vi "CH_LM Calibration Gain-Offset Dialog.vi"(0 "Meter Index":i32, 1 "Probe Type":T1, 5 "error in (no error)":errorcluster, 7 "Timeout / ms (3000)":i32=1000) -> (11 "Lock timed out":bool, 14 "Meter Index":i32, 15 "OK":bool, 16 "Thermopile Calibration":T5, 17 "Pyroelectric Calibration":T2, 18 "Optical Calibration":T4, 19 "error out":errorcluster)   [LabVIEW 2012, in "CH_LM.lvlib"]
doc: "This command stores gain and ADC offset correction data to the meter non-volatile memory. Different correction values are used for each input circuit and gain setting. See the Greenbuster TOP Theory of Operation for more information.\n\n<B>Note:</B> Error 100 will be raised if a valid password has not set since the last power off/on cycle."
uses:
  CH_LM.lvlib
  CH_LM Calibration Data Pyroelectric.ctl
  CH_LM Calibration Data Thermopile.ctl
  CH_LM Calibration Data Optical.ctl
  CH_LM ProbeType.ctl
  CH_LM Calibration Data.ctl
panel:
  in  "Cancel Button":bool
  out "Probe Type":T1
  in  "OK Button":bool
  in  "Optical Calibration":T4
  in  "Thermopile Calibration":T5
  in  "Pyroelectric Calibration":T2
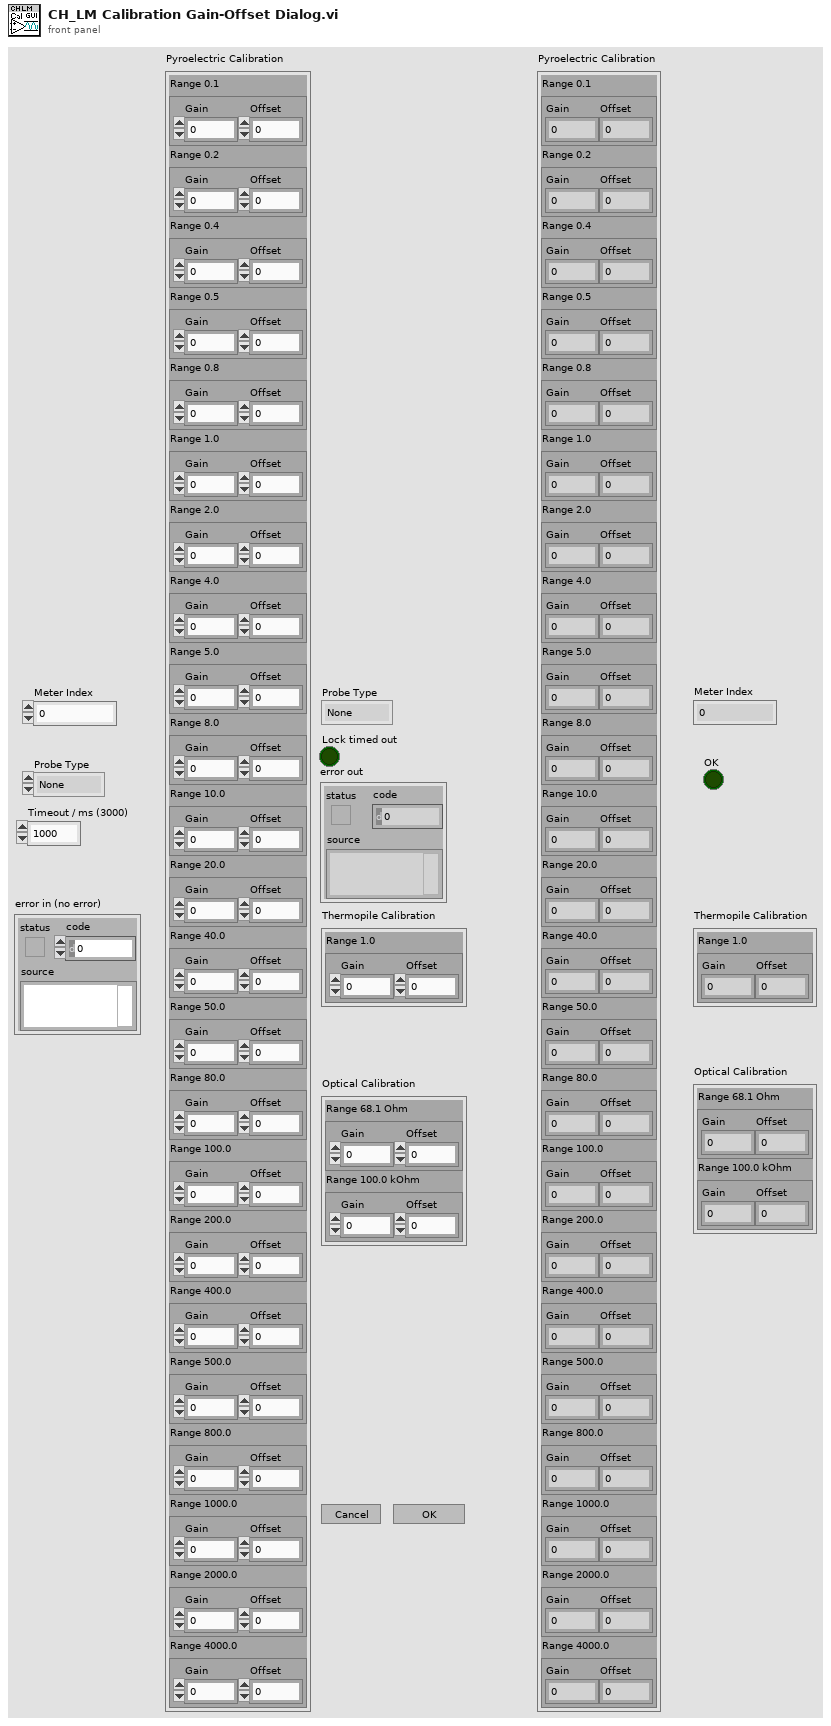
[diagram p1: front panel]
types:
  T1 = typedef "CH_LM.lvlib/CH_LM ProbeType.ctl" = enum16{"None", "Thermopile", "Pyroelectric", "Optical"}
  T2 = typedef "CH_LM.lvlib/CH_LM Calibration Data Pyroelectric.ctl" = cluster{"Range 0.1":T3, "Range 0.2":T3, "Range 0.4":T3, "Range 0.5":T3, "Range 0.8":T3, "Range 1.0":T3, "Range 2.0":T3, "Range 4.0":T3, "Range 5.0":T3, "Range 8.0":T3, "Range 10.0":T3, "Range 20.0":T3, "Range 40.0":T3, "Range 50.0":T3, "Range 80.0":T3, "Range 100.0":T3, "Range 200.0":T3, "Range 400.0":T3, "Range 500.0":T3, "Range 800.0":T3, "Range 1000.0":T3, "Range 2000.0":T3, "Range 4000.0":T3}
  T3 = typedef "CH_LM.lvlib/CH_LM Calibration Data.ctl" = cluster{"Gain":dbl, "Offset":dbl}
  T4 = typedef "CH_LM.lvlib/CH_LM Calibration Data Optical.ctl" = cluster{"Range 68.1 Ohm":T3, "Range 100.0 kOhm":T3}
  T5 = typedef "CH_LM.lvlib/CH_LM Calibration Data Thermopile.ctl" = cluster{"Range 1.0":T3}
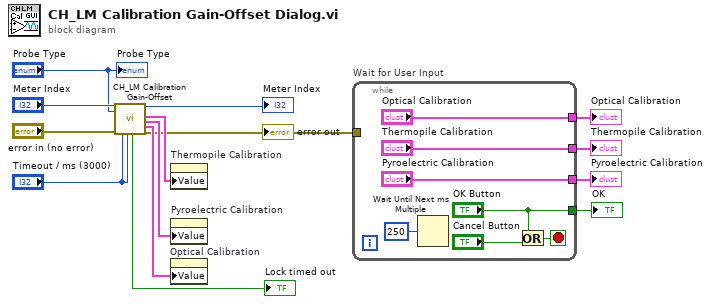
[diagram p0: block diagram]
diagram:
  n1 = call "CH_LM Calibration Gain-Offset.vi"("Meter Index"="Meter Index", "Probe Type"="Probe Type", "error in (no error)"="error in (no error)", "Timeout / ms (3000)"="Timeout / ms (3000)", "Lock Timeout / ms (1000)"="Timeout / ms (3000)") -> ("Lock timed out"=→"Lock timed out":bool, "Meter Index"=→"Meter Index":i32, "Thermopile Calibration"=w8:T5, "Pyroelectric Calibration"=w7:T2, "Optical Calibration"=w6:T4, "error out"=w2:errorcluster)  [unwired: 4 in, 5 out]
  "error out" <- w2
  n2 = property on="Thermopile Calibration" class="Clust (strict)"("Value"=w8) -> ()  [unwired: 2 in, 2 out]
  n3 = property on="Pyroelectric Calibration" class="Clust (strict)"("Value"=w7) -> ()  [unwired: 2 in, 2 out]
  n4 = property on="Optical Calibration" class="Clust (strict)"("Value"=w6) -> ()  [unwired: 2 in, 2 out]
  n5 = while "Wait for User Input" {
    tunnel: ["Optical Calibration"] -> w5
    tunnel: ["Thermopile Calibration"] -> w4
    tunnel: ["Pyroelectric Calibration"] -> w3
    tunnel: w2 -> [_]
    tunnel: ["OK Button"] -> w1
    stop <- w15 stop-if-true
    n6 = Wait Until Next ms Multiple(millisecond multiple=u32 250) -> ()  [unwired: 1 out]
    n7 = Or(x="OK Button", y="Cancel Button") -> (x .or. y?=w15:bool)
  }
  "Thermopile Calibration" <- w4
  "Pyroelectric Calibration" <- w3
  "Optical Calibration" <- w5
  "OK" <- w1
  "Probe Type" <- "Probe Type"
